vi "BNC555.evt call Chan Output.vi"(0 "i ref in":refnum<vi>, 2 "Generator Instance":string="N/A", 3 "Channel":i32(ring)=1 items=["System (To)", "Channel A", "Channel B", "Channel C", "Channel D", "Channel E", "Channel F", "Channel G", "Channel H"], 4 "Polarity (Normal)":enum16{"Normal", "Complement", "Inverted"}(ring), 5 "error in (no error)":errorcluster, 7 "Level (TTL)":enum16{"TTL", "Adjustable", "35 Volt"}(ring), 9 "Adjustable (5 Volts)":dbl=5.0 format="%.3p") -> (14 "i ref out":refnum<vi>, 19 "error out":errorcluster)   [LabVIEW 2014, in "BNC555.lvlib"]
doc: "This VI sends a simple event call to the wired BNC555."
uses:
  BNC555.lvlib
  CSCore/CSSystem/CoreLib/CoreLib.double 2 byte array.vi
  CSCore/CSSystem/CoreLib/CoreLib.short 2 byte array.vi
  CSCore/CSSystem/CoreLib/CoreLib.int 2 byte array.vi
  CSCore/CSSystem/CoreLib/CoreLib.lvlib
  CSCore/BaseProcess/BaseProcess.lvlib
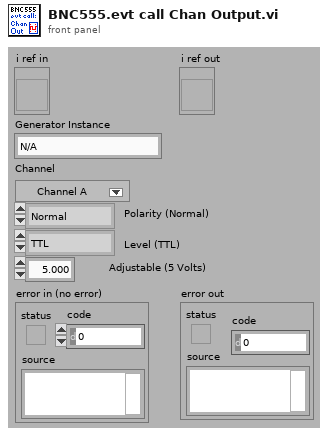
[diagram p1: front panel]
types:
  T1 = typedef "CoreDefs.rawDataType.ctl" = i8[]
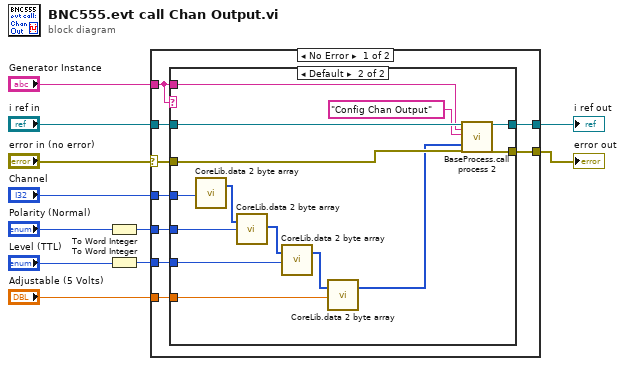
[diagram p0: block diagram]
diagram:
  n1 = To Word Integer(number="Polarity (Normal)") -> (16bit integer=w5:i16)
  n2 = To Word Integer(number="Level (TTL)") -> (16bit integer=w3:i16)
  n3 = case shown="No Error" "error in (no error)" {
    selector: "error in (no error)" -> [w17 w37]
    tunnel: [w20 w38] -> w10
    tunnel: [w19 w37] -> w9
    tunnel: "i ref in" -> [w18 w38]
    tunnel: "Generator Instance" -> [w16 _]
    tunnel: "Channel" -> [w15 _]
    tunnel: w5 -> [w14 _]
    tunnel: w3 -> [w13 _]
    tunnel: "Adjustable (5 Volts)" -> [w12 _]
    frame No Error {
      n4 = case shown="Default" w16 {
        tunnel: [w22 w36] -> w20
        tunnel: [w21 w35] -> w19
        tunnel: w18 -> [w22 w34]
        tunnel: w16 -> [_ w33]
        tunnel: w17 -> [w21 w31]
        tunnel: w15 -> [_ w30]
        tunnel: w14 -> [_ w29]
        tunnel: w13 -> [_ w24]
        tunnel: w12 -> [_ w23]
        frame "N/A" {
        }
        frame Default {
          n5 = call-poly "CoreLib.data 2 byte array.vi"("i32"=w30) -> ("byteArray out"=w28:T1)  [unwired: 18 in]
          n6 = call-poly "CoreLib.data 2 byte array.vi"("byteArray"=w28, "i16"=w29) -> ("byteArray out"=w26:T1)  [unwired: 17 in]
          n7 = call-poly "CoreLib.data 2 byte array.vi"("byteArray"=w26, "i16"=w24) -> ("byteArray out"=w27:T1)  [unwired: 17 in]
          n8 = call-poly "CoreLib.data 2 byte array.vi"("byteArray"=w27, "f64"=w23) -> ("byteArray out"=w25:T1)  [unwired: 17 in]
          n9 = call "BaseProcess.call process 2.vi"("i ref in"=w34, "Object"=w33, "Selector"="Config Chan Output", "Data"=w25, "error in (no error)"=w31) -> ("i ref out"=w36:refnum<vi>, "error out"=w35:errorcluster)  [unwired: 13 in]
        }
      }
    }
    frame Error {
    }
  }
  "error out" <- w9
  "i ref out" <- w10
